vi "Enable Defer Panel.vi"(8 "error in (no error)":errorcluster, 11 "Quick-GUI-Update in":refnum<class "Quick-GUI-Update.lvclass">) -> (0 "error out":errorcluster, 3 "Quick-GUI-Update out":refnum<class "Quick-GUI-Update.lvclass">)   [LabVIEW 2020, in "Quick-GUI-Update.lvclass"]
uses:
  Quick-GUI-Update.lvclass
  Quick-GUI-Update.lvclass/Quick-GUI-Update.ctl
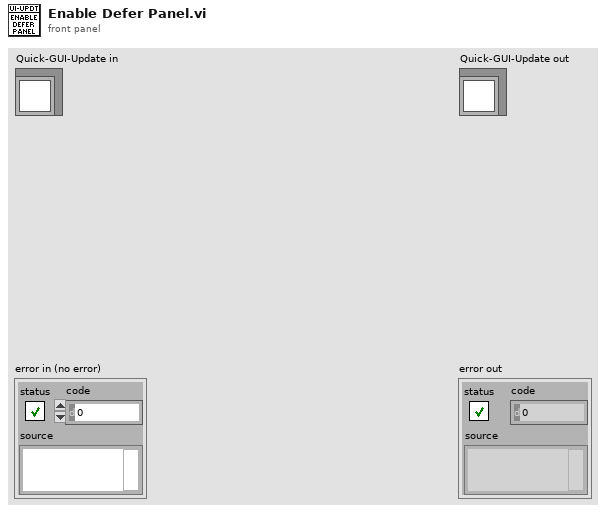
[diagram p1: front panel]
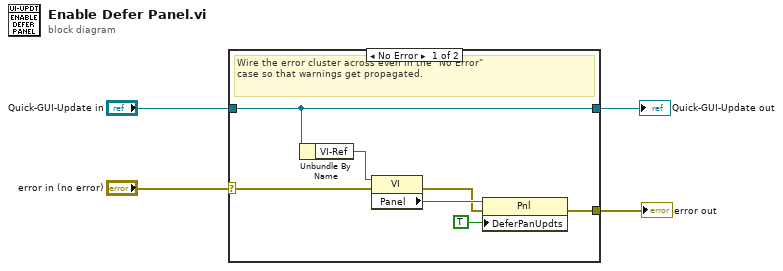
[diagram p0: block diagram]
diagram:
  n1 = case shown="No Error" "error in (no error)" {
    selector: "error in (no error)" -> [w8 w13]
    tunnel: [w5 w13] -> w3
    tunnel: [w10 w12] -> w1
    tunnel: "Quick-GUI-Update in" -> [w10 w12]
    frame No Error {
      # "Wire the error cluster across even in the \"No Error\"\ncase so that warnings get propagated."
      n2 = Unbundle By Name(w10) -> ("VI-Ref"=w9:refnum<vi>)
      n3 = property on="Property Node" class="VI"(reference=w9, error in=w8) -> (error out=w6:errorcluster, "Panel"=w7:refnum<vi>)  [unwired: 1 out]
      n4 = property on="Property Node" class="Pnl"(reference=w7, error in=w6, "DeferPanUpdts"=TRUE ("Defer Panel Updates")) -> (error out=w5:errorcluster)  [unwired: 1 out]
    }
    frame Error {
    }
  }
  "error out" <- w3
  "Quick-GUI-Update out" <- w1
